vi "CIF Manager UI.vi"() -> ()   [LabVIEW 2021, in "CIF Manager UI.lvlib"]
uses:
  CIF Manager UI.lvlib
  CIFManagerUI Class/Typedef/CIF_Manager_UI_Tab.ctl
  CIFManagerUI Class/Typedef/Core Manager UI References.ctl
  CIFManagerUI Class/CIF_Manager_UI.lvclass
  C:/Program Files/National Instruments/LabVIEW 2021/vi.lib/CIF Foundation/CIF Core/CIFUI/CIF_UI.lvclass
  CIFManagerUI Class/Typedef/Manager Subpanel Type.ctl
  <vilib>/CIF Foundation/CIF Core/CIFUI/Typedef/Core UI References.ctl
  <vilib>/CIF Foundation/CIF Core/CIFUI/CIF_UI.lvclass/CIF_UI.ctl
  CIFManagerUI Class/CIF_Manager_UI.lvclass/CIF_Manager_UI.ctl
  <vilib>/CIF Foundation/CIF Core/CIFUI/Utilities/Get Human Readable Error.vi
  <vilib>/CIF Foundation/CIF Utilities/Errors/Append Error Location.vi
  <vilib>/CIF Foundation/CIF Core/CIFUI/Accessors/Read Instrument Studio.vi
  <vilib>/CIF Foundation/CIF Core/CIFUI/UI Helpers/UI Element Update/Empty Table by Reference.vi
  <vilib>/CIF Foundation/CIF Core/CIFUI/UI Helpers/UI Element Update/Empty Tree by Reference.vi
  CIFManagerUI Class/Manager Functions/SubVIs/Initialize Manager Tab by Reference.vi
  <vilib>/CIF Foundation/CIF Utilities/Errors/Human Readable Error Message.vi
  <vilib>/CIF Foundation/CIF Core/CIFUI/CIF_UI.lvclass
panel:
  in  "Clear Local Error":bool
  out "System Errors":bool
  in  "EXIT":bool
  in  "Address":string="192.168.1.160"
  out "Connected":bool
  in  "Connection":bool
  in  "CIF Manager UI Tab":T1
  out "Local Error":string
  in  "Session Id":u64
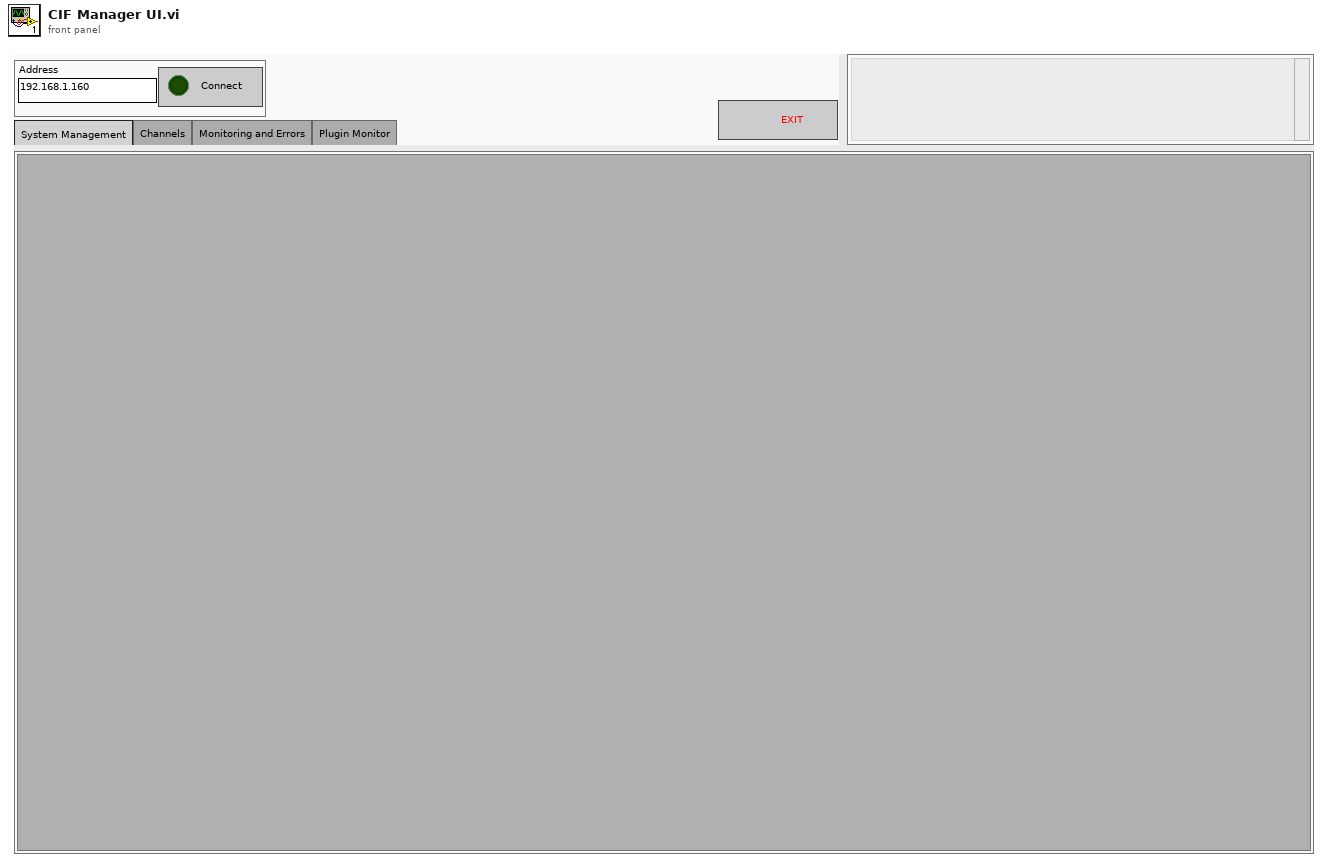
[diagram p1: front panel]
types:
  T1 = typedef "CIF_Manager_UI.lvclass/CIF_Manager_UI_Tab.ctl" = enum32{"System Management", "Channels", "Monitoring and Errors", "Plugin UI"}
  T2 = typedef "CIF_Manager_UI.lvclass/Core Manager UI References.ctl" = cluster{"Discovered Plugins":refnum<vi>, "Discovered Plugins Valid":bool, "Loaded Plugins":refnum<vi>, "Loaded Plugins Valid":bool, "Publisher Channels":refnum<vi>, "Publisher Channels Valid":bool, "Subscriber Channels":refnum<vi>, "Subscriber Channels Valid":bool, "Channel Connection":refnum<vi>, "Channel Connection Valid":bool, "New Plugin Load":refnum<vi>, "New Plugin Load Valid":bool, "Errors":refnum<vi>, "Errors Valid":bool, "Plugin to Abort":refnum<vi>, "Plugin to Abort Valid":bool, "CIF Manager Tab":refnum<vi>, "Manger Tab Valid":bool, "System Errors":refnum<vi>, "System Errors Valid":bool, "Plugin Selection":refnum<vi>, "Plugin Selection Valid":bool}
  T3 = typedef "CIF_Manager_UI.lvclass/Manager Subpanel Type.ctl" = enum16{"System", "Errors", "Channel", "Plugin"}
  T4 = typedef "CIF_UI.lvclass/Core UI References.ctl" = cluster{"Plugin Status":refnum<vi>, "Plugin Status Valid":bool, "Connection":refnum<vi>, "Connection Valid":bool, "Exit":refnum<vi>, "Exit Valid":bool, "Run Listen":refnum<vi>, "Run Listen Valid":bool, "Clear Local Error":refnum<vi>, "Clear Local Error Valid":bool, "Local Error":refnum<vi>, "Local Error Valid":bool}
  T5 = typedef "CIF_InstrumentStudio Plugin SDK.lvlib/Event Registration Refnum.ctl" = refnum<event-registration>
  T6 = cluster{"Event Refnum":T5, "Event Registration Refnum":refnum<event-registration>}
  T7 = typedef "CIF_Manager_UI_Tab.ctl" = enum32{"System Management", "Channels", "Monitoring and Errors", "Plugin UI"}
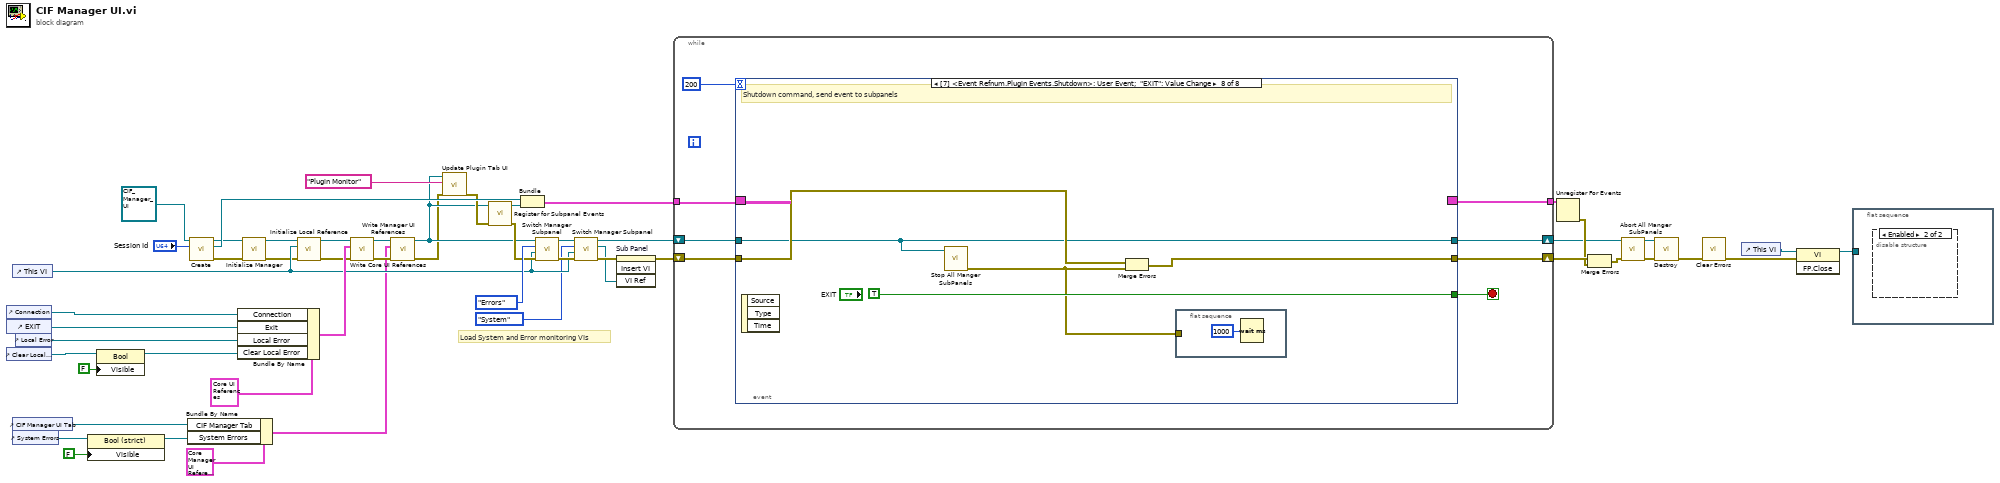
[diagram p0: block diagram]
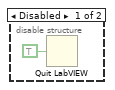
[diagram p2: hidden frame]
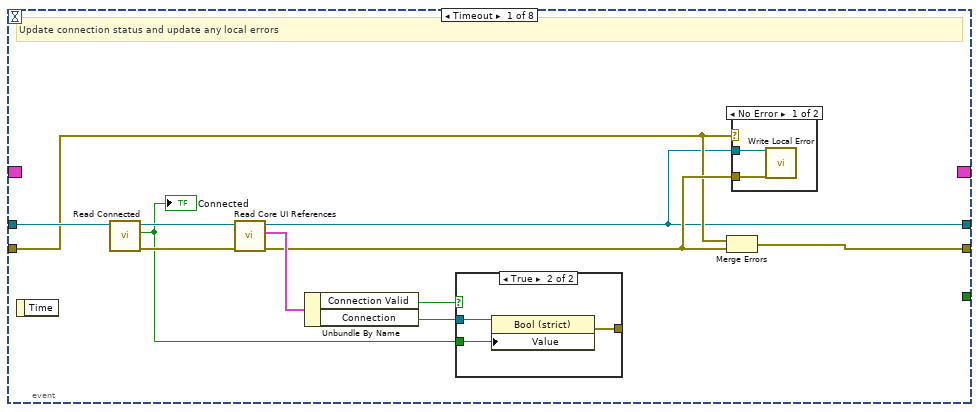
[diagram p3: hidden frame]
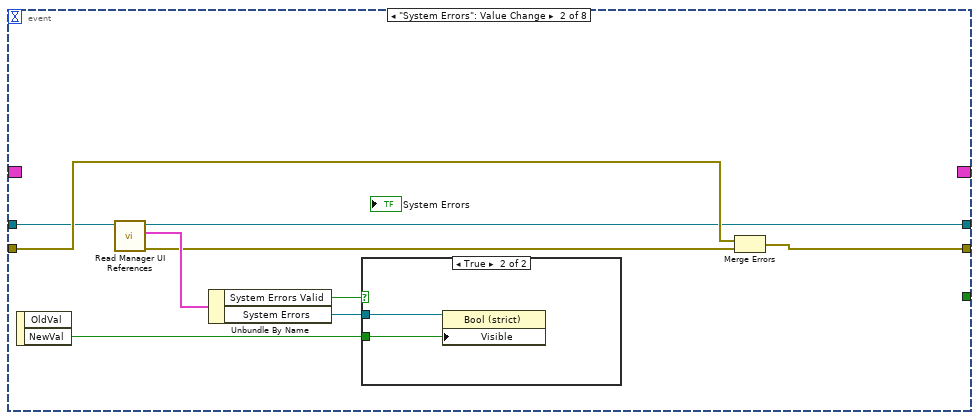
[diagram p6: hidden frame]
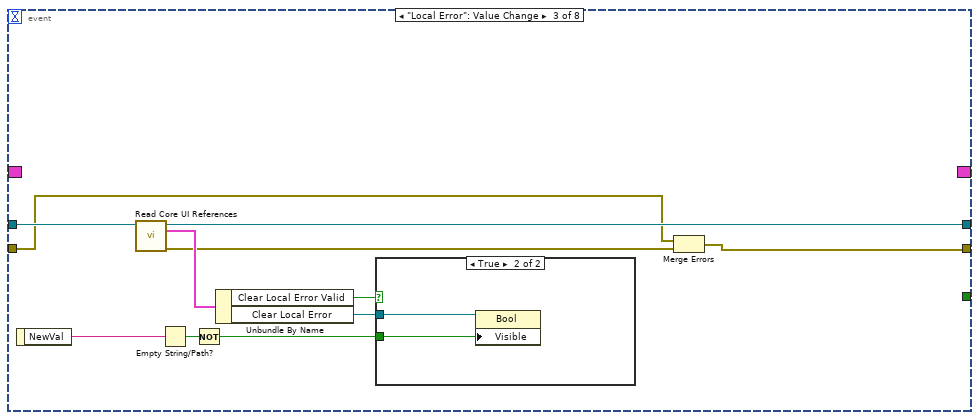
[diagram p8: hidden frame]
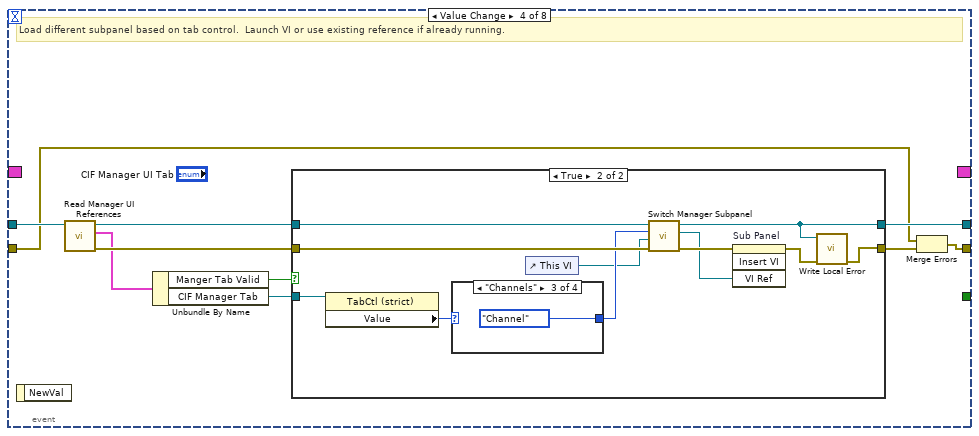
[diagram p10: hidden frame]
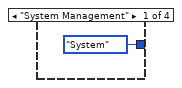
[diagram p12: hidden frame]
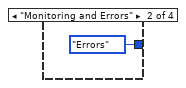
[diagram p13: hidden frame]
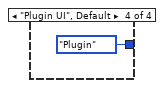
[diagram p14: hidden frame]
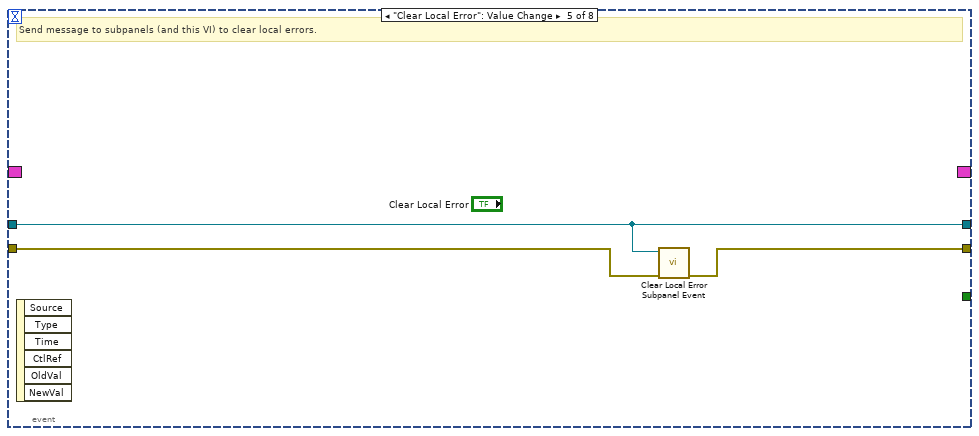
[diagram p15: hidden frame]
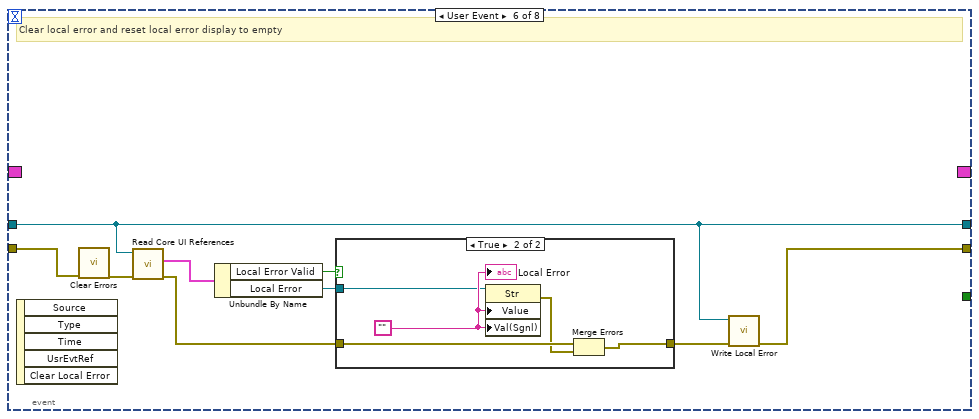
[diagram p16: hidden frame]
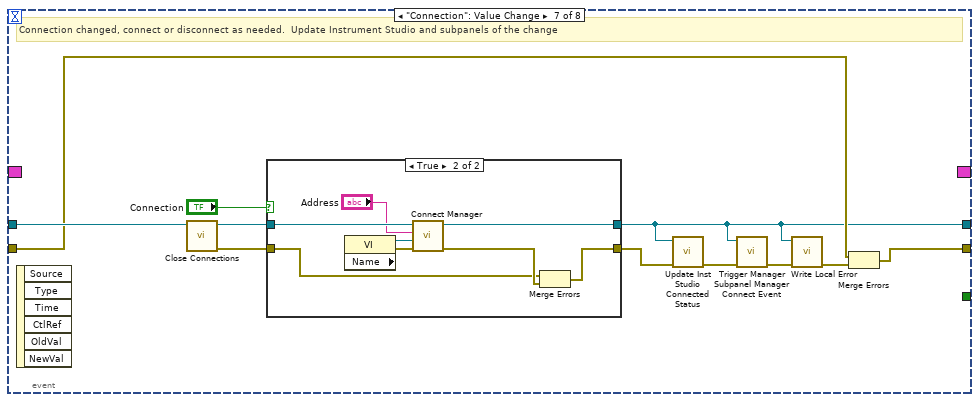
[diagram p18: hidden frame]
diagram:
  # "Load System and Error monitoring VIs"
  n1 = control-ref of="Connection"() -> (w48:refnum<vi>)
  n2 = control-ref of="EXIT"() -> (w49:refnum<vi>)
  n3 = control-ref of="Clear Local Error"() -> (w40:refnum<vi>)
  n4 = control-ref of="This VI"() -> (w21:refnum<vi>)
  n5 = control-ref of="CIF Manager UI Tab"() -> (w16:refnum<vi>)
  n6 = control-ref of="System Errors"() -> (w37:refnum<vi>)
  n7 = control-ref of="Local Error"() -> (w39:refnum<vi>)
  n8 = property class="Bool (strict)"(reference=w37, "Visible"=FALSE) -> (reference out=w17:refnum<vi>)  [unwired: 1 in, 1 out]
  n9 = property class="Bool"(reference=w40, "Visible"=FALSE) -> (reference out=w38:refnum<vi>)  [unwired: 1 in, 1 out]
  n10 = Bundle By Name(cluster=T2 {"Discovered Plugins"=refnum, "Discovered Plugins Valid"=FALSE, "Loaded Plugins"=refnum, "Loaded Plugins Valid"=FALSE, "Publisher Channels"=refnum, "Publisher Channels Valid"=FALSE, "Subscriber Channels"=refnum, "Subscriber Channels Valid"=FALSE, "Channel Connection"=refnum, "Channel Connection Valid"=FALSE, "New Plugin Load"=refnum, "New Plugin Load Valid"=FALSE, "Errors"=refnum, "Errors Valid"=FALSE, "Plugin to Abort"=refnum, "Plugin to Abort Valid"=FALSE, "CIF Manager Tab"=refnum, "Manger Tab Valid"=FALSE, "System Errors"=refnum, "System Errors Valid"=FALSE, "Plugin Selection"=refnum, "Plugin Selection Valid"=FALSE} ("Manager UI References"), "CIF Manager Tab"=w16, "System Errors"=w17) -> (w9:T2)
  n11 = call <vilib>:"Create.vi"("Session Id"="Session Id", "CIF_UI in"=refnum<class "CIF_Manager_UI.lvclass"> refnum ("CIF_Manager_UI.lvclass")) -> ("error out"=w3:errorcluster, "Event Refnum"=w46:T5, "CIF_UI out"=w4:refnum<class "CIF_Manager_UI.lvclass">)  [unwired: 7 in]
  n12 = Bundle By Name(cluster=T4 {"Plugin Status"=refnum, "Plugin Status Valid"=FALSE, "Connection"=refnum, "Connection Valid"=FALSE, "Exit"=refnum, "Exit Valid"=FALSE, "Run Listen"=refnum, "Run Listen Valid"=FALSE, "Clear Local Error"=refnum, "Clear Local Error Valid"=FALSE, "Local Error"=refnum, "Local Error Valid"=FALSE} ("UI References"), "Connection"=w48, "Exit"=w49, "Local Error"=w39, "Clear Local Error"=w38) -> (w50:T4)
  n13 = call "Initialize Manager.vi"("error in (no error)"=w3, "CIF_Manager_UI in"=w4) -> ("error out"=w1:errorcluster, "CIF_Manager_UI out"=w2:refnum<class "CIF_Manager_UI.lvclass">)  [unwired: 8 in]
  n14 = call <vilib>:"Initialize Local Reference.vi"("error in (no error)"=w1, "This VI"=w21, "CIF_UI in"=w2) -> ("error out"=w43:errorcluster, "CIF_UI out"=w42:refnum<class "CIF_Manager_UI.lvclass">)  [unwired: 7 in]
  n15 = call <vilib>:"Write Core UI References.vi"("error in (no error)"=w43, "UI References"=w50, "CIF_UI in"=w42) -> ("error out"=w12:errorcluster, "CIF_UI out"=w13:refnum<class "CIF_Manager_UI.lvclass">)  [unwired: 7 in]
  n16 = call "Write Manager UI References.vi"("error in (no error)"=w12, "Manager UI References"=w9, "CIF_UI in"=w13) -> ("error out"=w10:errorcluster, "CIF_UI out"=w11:refnum<class "CIF_Manager_UI.lvclass">)  [unwired: 7 in]
  n17 = call "Update Plugin Tab UI.vi"("error in (no error)"=w10, "Plugin Name"="Plugin Monitor", "CIF_UI in"=w11) -> ("error out"=w28:errorcluster)  [unwired: 8 in]
  n18 = call <vilib>:"Register for Subpanel Events.vi"("error in (no error)"=w28, "CIF_UI in"=w11) -> ("error out"=w26:errorcluster, "Event Registration Refnum"=w47:refnum<event-registration>)  [unwired: 8 in]
  n19 = Bundle("Event Refnum"=w46, "Event Registration Refnum"=w47) -> (w45:T6)  [unwired: 1 in]
  n20 = call "Switch Manager Subpanel.vi"("error in (no error)"=w26, "Calling VI"=w21, "Subpanel Type"=Manager_Subpanel_Type."Errors", "CIF_UI in"=w11) -> ("error out"=w22:errorcluster, "CIF_UI out"=w25:refnum<class "CIF_Manager_UI.lvclass">)  [unwired: 5 in, 1 out]
  n21 = call "Switch Manager Subpanel.vi"("error in (no error)"=w22, "Calling VI"=w21, "Subpanel Type"=Manager_Subpanel_Type."System", "CIF_UI in"=w25) -> ("error out"=w23:errorcluster, "VI Reference"=w19:refnum<vi>, "CIF_UI out"=w24:refnum<class "CIF_Manager_UI.lvclass">)  [unwired: 5 in]
  n22 = invoke on="Sub Panel" class="SubPnl" method="Insert VI"(error in=w23, "VI Ref"=w19) -> (error out=w44:errorcluster)  [unwired: 2 in, 3 out]
  n23 = while {
    shift-right: [w56] -> w8
    shift-left: w24 -> [w58]
    shift-right: [w53] -> w34
    shift-left: w44 -> [w57]
    tunnel: w45 -> [w55]
    tunnel: [w54] -> w41
    stop <- w59 stop-if-true
    n24 = event shown="[7] <Event Refnum.Plugin Events.Shutdown>: User Event;  \"EXIT\": Value Change" {
      selector: w55 -> [_ _ _ _ _ _ _ _]
      dyn-events: [_ _ _ _ _ _ _ _] -> w54
      timeout: 200 -> [_ _ _ _ _ _ _ _]
      tunnel: [_ _ _ _ _ _ _ TRUE] -> w59
      tunnel: w58 -> [w71 w80 w95 w109 w130 w131 w156 w168]
      tunnel: w57 -> [w63 w82 w89 w101 w129 w138 w150 w170]
      tunnel: [w61 w81 w88 w102 w128 w132 w149 w169] -> w53
      tunnel: [w62 w78 w94 w110 w130 w131 w146 w168] -> w56
      event Timeout {
        # "Update connection status and update any local errors"
        n25 = event-data() -> ()  [unwired: 1 in, 1 out]
        n26 = call <vilib>:"Read Connected.vi"("CIF_UI in"=w71) -> ("error out"=w69:errorcluster, "Connected"=w65:bool, "CIF_UI out"=w70:refnum<class "CIF_Manager_UI.lvclass">)  [unwired: 8 in]
        "Connected" <- w65
        n27 = call <vilib>:"Read Core UI References.vi"("error in (no error)"=w69, "CIF_UI in"=w70) -> ("error out"=w64:errorcluster, "UI References"=w66:T4, "CIF_UI out"=w62:refnum<class "CIF_Manager_UI.lvclass">)  [unwired: 7 in]
        n28 = Unbundle By Name(w66) -> ("Connection Valid"=w68:bool, "Connection"=w67:refnum<vi>)
        n29 = case shown="True" w68 {
          tunnel: w67 -> [_ w76]
          tunnel: w65 -> [_ w75]
          tunnel: [_ w74] -> _
          frame False {
          }
          frame True {
            n30 = property class="Bool (strict)"(reference=w76, "Value"=w75) -> (error out=w74:errorcluster)  [unwired: 1 in, 1 out]
          }
        }
        n31 = Merge Errors(w63, w64) -> (w61:errorcluster)
        n32 = case shown="No Error" w63 {
          tunnel: w62 -> [w73 _]
          tunnel: w64 -> [w72 _]
          frame No Error {
            n33 = call <vilib>:"Write Local Error.vi"("error in (no error)"=w72, "CIF_UI in"=w73) -> ()  [unwired: 9 in, 1 out]
          }
          frame Error {
          }
        }
      }
      event "System Errors": Value Change {
        n34 = event-data() -> ("NewVal"=w83:bool)  [unwired: 1 in, 1 out]
        n35 = call "Read Manager UI References.vi"("CIF_UI in"=w80) -> ("error out"=w77:errorcluster, "UI References"=w79:T2, "CIF_UI out"=w78:refnum<class "CIF_Manager_UI.lvclass">)  [unwired: 8 in]
        n36 = Unbundle By Name(w79) -> ("System Errors Valid"=w85:bool, "System Errors"=w84:refnum<vi>)
        n37 = case shown="True" w85 {
          tunnel: w84 -> [_ w87]
          tunnel: w83 -> [_ w86]
          frame False {
          }
          frame True {
            n38 = property class="Bool (strict)"(reference=w87, "Visible"=w86) -> ()  [unwired: 1 in, 2 out]
          }
        }
        n39 = Merge Errors(w82, w77) -> (w81:errorcluster)
      }
      event "Local Error": Value Change {
        n40 = event-data() -> ("NewVal"=w93:string)  [unwired: 1 in]
        n41 = call <vilib>:"Read Core UI References.vi"("CIF_UI in"=w95) -> ("error out"=w90:errorcluster, "UI References"=w98:T4, "CIF_UI out"=w94:refnum<class "CIF_Manager_UI.lvclass">)  [unwired: 8 in]
        n42 = Empty String/Path?(string/path=w93) -> (empty?=w92:bool)
        n43 = Not(x=w92) -> (.not. x?=w91:bool)
        n44 = Unbundle By Name(w98) -> ("Clear Local Error Valid"=w97:bool, "Clear Local Error"=w96:refnum<vi>)
        n45 = case shown="True" w97 {
          tunnel: w96 -> [_ w100]
          tunnel: w91 -> [_ w99]
          frame False {
          }
          frame True {
            n46 = property class="Bool"(reference=w100, "Visible"=w99) -> ()  [unwired: 1 in, 2 out]
          }
        }
        n47 = Merge Errors(w89, w90) -> (w88:errorcluster)
      }
      event Value Change {
        # "Load different subpanel based on tab control.  Launch VI or use existing reference if already running."
        n48 = event-data() -> ()  [unwired: 1 in, 1 out]
        n49 = call "Read Manager UI References.vi"("CIF_UI in"=w109) -> ("error out"=w107:errorcluster, "UI References"=w106:T2, "CIF_UI out"=w108:refnum<class "CIF_Manager_UI.lvclass">)  [unwired: 8 in]
        n50 = Unbundle By Name(w106) -> ("Manger Tab Valid"=w104:bool, "CIF Manager Tab"=w105:refnum<vi>)
        n51 = case shown="True" w104 {
          tunnel: [w112 w115] -> w110
          tunnel: [w111 w113] -> w103
          tunnel: w108 -> [w112 w121]
          tunnel: w107 -> [w111 w120]
          tunnel: w105 -> [_ w119]
          frame False {
          }
          frame True {
            n52 = property class="TabCtl (strict)"(reference=w119) -> ("Value"=w118:T7)  [unwired: 1 in, 2 out]
            n53 = case shown="\"Channels\"" w118 {
              tunnel: [Manager_Subpanel_Type."System" ("Subpanel Type") Manager_Subpanel_Type."Errors" ("Subpanel Type") Manager_Subpanel_Type."Channel" ("Subpanel Type") Manager_Subpanel_Type."Plugin" ("Subpanel Type")] -> w117
              frame "System Management" {
              }
              frame "Monitoring and Errors" {
              }
              frame "Channels" {
              }
              frame "Plugin UI", Default {
              }
            }
            n54 = control-ref of="This VI"() -> (w116:refnum<vi>)
            n55 = call "Switch Manager Subpanel.vi"("error in (no error)"=w120, "Calling VI"=w116, "Subpanel Type"=w117, "CIF_UI in"=w121) -> ("error out"=w123:errorcluster, "VI Reference"=w122:refnum<vi>, "CIF_UI out"=w115:refnum<class "CIF_Manager_UI.lvclass">)  [unwired: 5 in]
            n56 = invoke on="Sub Panel" class="SubPnl" method="Insert VI"(error in=w123, "VI Ref"=w122) -> (error out=w114:errorcluster)  [unwired: 2 in, 3 out]
            n57 = call <vilib>:"Write Local Error.vi"("error in (no error)"=w114, "CIF_UI in"=w115) -> ("error out"=w113:errorcluster)  [unwired: 9 in]
          }
        }
        n58 = Merge Errors(w101, w103) -> (w102:errorcluster)
      }
      event "Clear Local Error": Value Change {
        # "Send message to subpanels (and this VI) to clear local errors."
        n59 = event-data() -> ()  [unwired: 1 in, 6 out]
        n60 = call <vilib>:"Clear Local Error Subpanel Event.vi"("error in (no error)"=w129, "CIF_UI in"=w130) -> ("error out"=w128:errorcluster)  [unwired: 9 in]
      }
      event User Event {
        # "Clear local error and reset local error display to empty"
        n61 = event-data() -> ()  [unwired: 1 in, 5 out]
        n62 = call <vilib>:"Clear Errors.vi"("error in (no error)"=w138) -> ("error out"=w139:errorcluster)  [unwired: 5 in, 1 out]
        n63 = call <vilib>:"Read Core UI References.vi"("error in (no error)"=w139, "CIF_UI in"=w131) -> ("error out"=w136:errorcluster, "UI References"=w137:T4)  [unwired: 7 in, 1 out]
        n64 = Unbundle By Name(w137) -> ("Local Error Valid"=w135:bool, "Local Error"=w134:refnum<vi>)
        n65 = case shown="True" w135 {
          tunnel: w134 -> [_ w141]
          tunnel: w136 -> [w140 w145]
          tunnel: [w140 w143] -> w133
          frame False {
          }
          frame True {
            w142 = ""
            n66 = property class="Str"(reference=w141, "Value"=w142, "Val(Sgnl)"=w142) -> (error out=w144:errorcluster)  [unwired: 1 in, 1 out]
            n67 = Merge Errors(w145, w144) -> (w143:errorcluster)
            "Local Error" <- w142
          }
        }
        n68 = call <vilib>:"Write Local Error.vi"("error in (no error)"=w133, "CIF_UI in"=w131) -> ("error out"=w132:errorcluster)  [unwired: 9 in]
      }
      event "Connection": Value Change {
        # "Connection changed, connect or disconnect as needed.  Update Instrument Studio and subpanels of the change"
        n69 = event-data() -> ()  [unwired: 1 in, 6 out]
        n70 = call <vilib>:"Close Connections.vi"("CIF_UI in"=w156) -> ("error out"=w155:errorcluster, "CIF_UI out"=w154:refnum<class "CIF_Manager_UI.lvclass">)  [unwired: 9 in]
        n71 = case shown="True" "Connection" {
          tunnel: [w158 w163] -> w146
          tunnel: [w157 w162] -> w152
          tunnel: w155 -> [w157 w161]
          tunnel: w154 -> [w158 w160]
          frame False {
          }
          frame True {
            n72 = property class="VI" props=["Name"]() -> (reference out=w166:refnum<vi>, error out=w165:errorcluster)  [unwired: 2 in, 1 out]
            n73 = call <vilib>:"Connect Manager.vi"("error in (no error)"=w165, "VI Reference"=w166, "Address"="Address", "CIF_UI in"=w160) -> ("error out"=w164:errorcluster, "CIF_UI out"=w163:refnum<class "CIF_Manager_UI.lvclass">)  [unwired: 6 in]
            n74 = Merge Errors(w161, w164) -> (w162:errorcluster)
          }
        }
        n75 = call <vilib>:"Update Inst Studio Connected Status.vi"("error in (no error)"=w152, "CIF_UI in"=w146) -> ("error out"=w148:errorcluster)  [unwired: 9 in]
        n76 = call "Trigger Manager Subpanel Manager Connect Event.vi"("error in (no error)"=w148, "CIF_Manager_UI in"=w146) -> ("error out"=w147:errorcluster)  [unwired: 9 in]
        n77 = call <vilib>:"Write Local Error.vi"("error in (no error)"=w147, "CIF_UI in"=w146) -> ("error out"=w151:errorcluster)  [unwired: 9 in]
        n78 = Merge Errors(w150, w151) -> (w149:errorcluster)
      }
      event User Event; "EXIT": Value Change {
        # "Shutdown command, send event to subpanels"
        n79 = event-data() -> ()  [unwired: 1 in, 3 out]
        n80 = call "Stop All Manger SubPanels.vi"("CIF_UI in"=w168) -> ("error out"=w167:errorcluster)  [unwired: 10 in]
        n81 = Merge Errors(w170, w167) -> (w169:errorcluster)
        n82 = flat-sequence {
          tunnel: w167 -> [_]
          frame #0 {
            n83 = Wait (ms)(milliseconds to wait=u32 1000) -> ()  [unwired: 1 out]
          }
        }
      }
    }
  }
  n84 = Unregister For Events(event registration refnum=w41) -> (error out=w33:errorcluster)  [unwired: 1 in]
  n85 = Merge Errors(w34, w33) -> (w5:errorcluster)
  n86 = call "Abort All Manger SubPanels.vi"("error in (no error)"=w5, "CIF_UI in"=w8) -> ("error out"=w7:errorcluster, "CIF_UI out"=w6:refnum<class "CIF_Manager_UI.lvclass">)  [unwired: 8 in]
  n87 = call <vilib>:"Destroy.vi"("error in (no error)"=w7, "CIF_UI in"=w6) -> ("error out"=w36:errorcluster)  [unwired: 8 in, 1 out]
  n88 = call <vilib>:"Clear Errors.vi"("error in (no error)"=w36) -> ("error out"=w35:errorcluster)  [unwired: 5 in, 1 out]
  n89 = control-ref of="This VI"() -> (w32:refnum<vi>)
  n90 = invoke class="VI" method="FP.Close"(reference=w32, error in=w35) -> (reference out=w31:refnum<vi>)  [unwired: 1 in, 2 out]
  n91 = flat-sequence {
    tunnel: w31 -> [_]
    frame #0 {
      n92 = disable-structure shown="Enabled" {
        frame Disabled {
          n93 = Quit LabVIEW(quit? (T)=TRUE) -> ()
        }
        frame Enabled {
        }
      }
    }
  }
